vi "ReadEyeFile.vi"(0 "new file path":path=path "C:/WINDOWS/DESKTOP/rri.eye", 6 "Header format":u16(ring) items=["Riverside Format", "Ron Linear"]) -> (10 "new path out":path, 12 "1-D data":i16[](array[numeric]), 13 "2-D data array":i16[][](array[numeric]), 14 "# lines per scan":u16, 15 "# rf points per line":u16, 16 "sample rate MHz":u16, 17 "sector scan angle":sgl format="%.2f", 18 "delay":sgl format="%.2f", 19 "pivot distance":sgl format="%.2f")   [LabVIEW 2022 SP3]
uses:
  ADInfo.vi
panel:
  out "error out":errorcluster
  in  "Correct Delay?":bool=TRUE
  out "Head length":i16
  out "file size (bytes)":i32
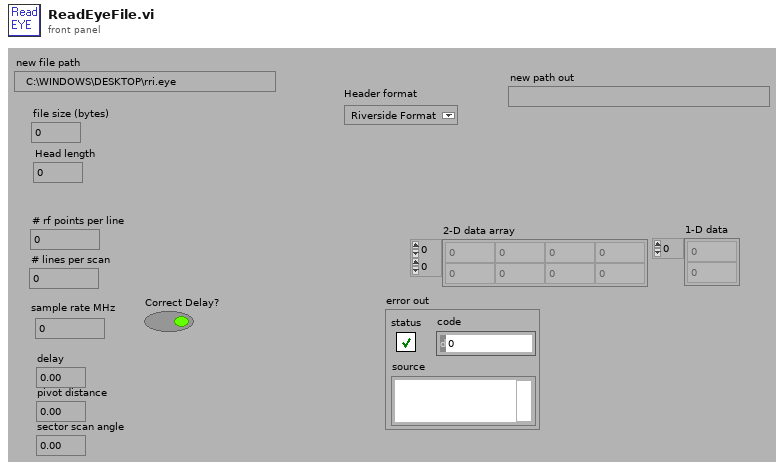
[diagram p1: front panel]
types:
  T1 = enum16{"big-endian, network order", "native, host order", "little-endian"}
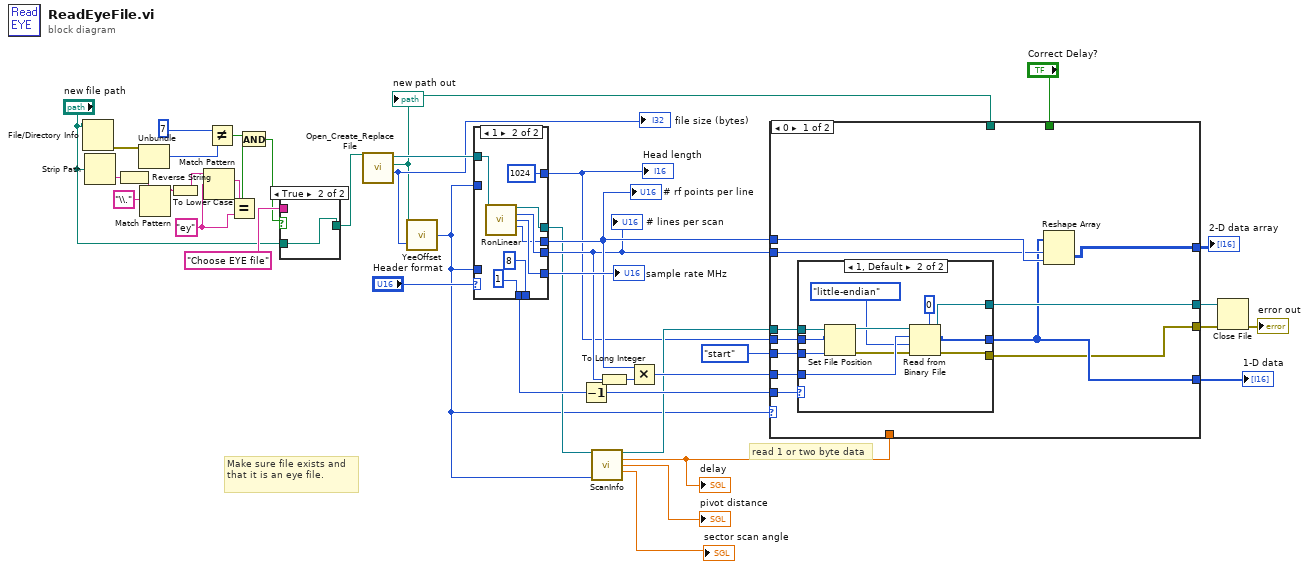
[diagram p0: block diagram]
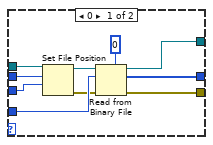
[diagram p2: hidden frame]
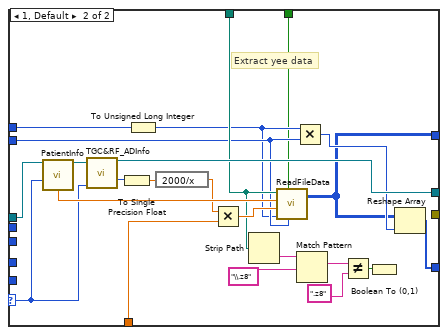
[diagram p3: hidden frame]
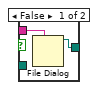
[diagram p4: hidden frame]
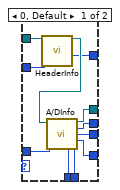
[diagram p5: hidden frame]
diagram:
  w7 = "ey"
  # "Make sure file exists and that it is an eye file."
  # "read 1 or two byte data"
  n1 = File/Directory Info(path="new file path") -> (error out=w24:errorcluster)  [unwired: 1 in, 6 out]
  n2 = Strip Path(path="new file path") -> (name=w29:string)  [unwired: 1 out]
  n3 = Reverse String(1:w29) -> (0:w22:string)
  n4 = Unbundle(w24) -> ("code"=w23:i32)  [unwired: 2 out]
  n5 = Match Pattern(string=w22, regular expression="\\.") -> (before substring=w21:string)  [unwired: 4 out]
  n6 = To Lower Case(string=w21) -> (all lower case string=w8:string)
  n7 = Match Pattern(string=w8, regular expression=w7) -> (match substring=w6:string)  [unwired: 4 out]
  n8 = Not Equal?(x=7, y=w23) -> (x != y?=w26:bool)
  n9 = Equal?(x=w6, y=w7) -> (x = y?=w28:bool)
  n10 = And(x=w26, y=w28) -> (x .and. y?=w25:bool)
  n11 = case shown="True" w25 {
    tunnel: [w43 w44] -> w32
    tunnel: "new file path" -> [_ w44]
    tunnel: "Choose EYE file" -> [w42 _]
    frame False {
      n12 = File Dialog(7:w42) -> (3:w43:path)  [unwired: 1 in, 8 out]
    }
    frame True {
    }
  }
  n13 = call <vilib>:"Open_Create_Replace File.vi"("file path"=w32) -> ("file size (bytes)"=w19:i32, "new file path"=w12:path, "refnum"=w38:refnum<file>)  [unwired: 5 in, 3 out]
  "file size (bytes)" <- w19
  "new path out" <- w12
  n14 = call "YeeOffset.vi"("file size (bytes)"=w19, "new file path"=w12) -> ("Numeric"=w13:i32)
  n15 = case shown="1" "Header format" {
    tunnel: [w55 w59] -> w40
    tunnel: w38 -> [w54 w61]
    tunnel: [w53 w57] -> w18
    tunnel: [w52 w63] -> w17
    tunnel: [w50 w62] -> w16
    tunnel: [w49 1024] -> w3
    tunnel: [w48 1] -> w33
    tunnel: w13 -> [w47 _]
    tunnel: w13 -> [w46 _]
    tunnel: [w45 8] -> _
    frame 0, Default {
      n16 = call "HeaderInfo.vi"("refnum"=w54, "offset"=w47) -> ("dup refnum"=w51:refnum<file>, "header length"=w49:i16)  [unwired: 12 out]
      n17 = call "A/DInfo.vi"("refnum"=w51, "offset"=w46) -> ("dup refnum"=w50:refnum<file>, "# rf points per line"=w53:u16, "# lines per scan"=w52:u16, "sample rate MHz"=w55:u16, "# bytes per A/D"=w48:u16, "# A/D bits"=w45:u16)  [unwired: 8 out]
    }
    frame 1 {
      n18 = call "RonLinear.vi"("refnum"=w61) -> ("refnum out"=w62:refnum<file>, "# lines per scan"=w63:i32, "sample rate"=w59:u16, "# rf points per line"=w57:u16)  [unwired: 11 out]
    }
  }
  "# rf points per line" <- w18
  "Head length" <- w3
  "# lines per scan" <- w17
  "sample rate MHz" <- w40
  n19 = Decrement(x=w33) -> (x-1=w34:i32)
  n20 = call "ScanInfo.vi"("refnum"=w16, "offset"=w13) -> ("dup refnum"=w14:refnum<file>, "delay"=w10:sgl, "pivot distance"=→"pivot distance":sgl, "sector scan angle"=→"sector scan angle":sgl)  [unwired: 10 out]
  "delay" <- w10
  n21 = To Long Integer(number=w17) -> (32bit integer=w36:i32)
  n22 = Multiply(x=w18, y=w36) -> (x*y=w37:i32)
  n23 = case shown="0" w13 {
    selector: w13 -> [_ w109]
    tunnel: enum16{"start", "end", "current"}."start" ("pos mode (0:2)") -> [w74 _]
    tunnel: w37 -> [w73 _]
    tunnel: w34 -> [w68 _]
    tunnel: w18 -> [w72 w102]
    tunnel: w17 -> [w71 w101]
    tunnel: w14 -> [w70 w118]
    tunnel: w12 -> [_ w108]
    tunnel: [w69 w110] -> w11
    tunnel: [w65 w96] -> w4
    tunnel: w10 -> [_ w112]
    tunnel: [w67 w103] -> w9
    tunnel: "Correct Delay?" -> [_ w97]
    tunnel: w3 -> [w66 _]
    tunnel: [w64 _] -> w2
    frame 0 {
      n24 = case shown="1, Default" w68 {
        tunnel: w74 -> [w83 w92]
        tunnel: [w79 w86] -> w67
        tunnel: w73 -> [w82 w93]
        tunnel: w70 -> [w81 w95]
        tunnel: w66 -> [w80 w88]
        tunnel: [w78 w91] -> w69
        tunnel: [w75 w85] -> w64
        frame 0 {
          n25 = Set File Position(offset (in bytes) (0)=w80, refnum=w81, from (0:start)=w83) -> (refnum out=w77:refnum<file>, error out=w76:errorcluster)  [unwired: 1 in]
          n26 = Read from Binary File(5:i8 0, 8:w76, 10:w82, 11:w77) -> (0:w75:errorcluster, 2:w79:i8[], 3:w78:refnum<file>)  [unwired: 3 out]
        }
        frame 1, Default {
          n27 = Set File Position(offset (in bytes) (0)=w88, refnum=w95, from (0:start)=w92) -> (refnum out=w90:refnum<file>, error out=w89:errorcluster)  [unwired: 1 in]
          n28 = Read from Binary File(5:i16 0, 8:w89, 9:T1."little-endian" ("byte order (0:big-endian, network order)"), 10:w93, 11:w90) -> (0:w85:errorcluster, 2:w86:i16[], 3:w91:refnum<file>)  [unwired: 2 out]
        }
      }
      n29 = Reshape Array(w67, w71, w72) -> (w65:i16[][])
    }
    frame 1, Default {
      # "Extract yee data"
      n30 = call "PatientInfo.vi"("refnum"=w118, "offset"=w109) -> ("dup refnum"=w117:refnum<file>, "PSA"=w115:sgl)  [unwired: 12 out]
      n31 = call "TGC&RF_ADInfo.vi"("refnum"=w117, "offset"=w109) -> ("dup refnum"=w110:refnum<file>, "c speed"=w116:i16)  [unwired: 12 out]
      n32 = To Single Precision Float(number=w116) -> (single precision float=w114:sgl)
      n33 = To Unsigned Long Integer(number=w102) -> (unsigned 32bit integer=w100:u32)
      n34 = expression code="2000/x"(w114) -> (w113:sgl)
      n35 = Multiply(x=w113, y=w112) -> (x*y=w111:sgl)
      n36 = Strip Path(path=w108) -> (name=w107:string)  [unwired: 1 out]
      n37 = call "ReadFileData.vi"("RF lines"=w101, "Correct Delay?"=w97, "RF Points"=w100, "Delay mics"=w111, "yee delay"=w115, "File Path"=w108) -> ("Data"=w96:i16[][])  [unwired: 1 out]
      n38 = Multiply(x=w100, y=w101) -> (x*y=w98:u32)
      n39 = Match Pattern(string=w107, regular expression="\\.z8") -> (match substring=w106:string)  [unwired: 4 out]
      n40 = Not Equal?(x=w106, y=".z8") -> (x != y?=w104:bool)
      n41 = Boolean To (0,1)(Boolean=w104) -> ()  [unwired: 1 out]
      n42 = Reshape Array(w96, w98) -> (w103:i16[])
    }
  }
  "2-D data array" <- w4
  "1-D data" <- w9
  n43 = Close File(refnum=w11, error in=w2) -> (error out=→"error out":errorcluster)  [unwired: 1 out]
